vi "RecrystalliseSendAHKcmd.vi"(8 "error in (no error)":errorcluster, 11 "Enum":enum16{"low", "high"}(ring)) -> (0 "error out":errorcluster)   [LabVIEW 2017]
panel:
  out "timed out?":bool
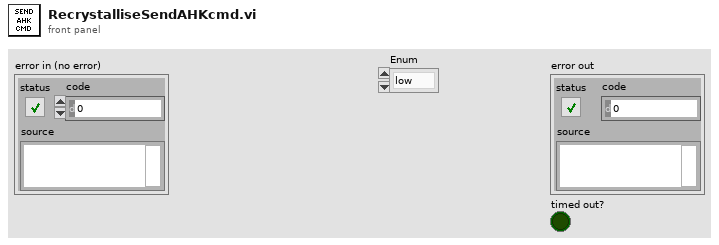
[diagram p1: front panel]
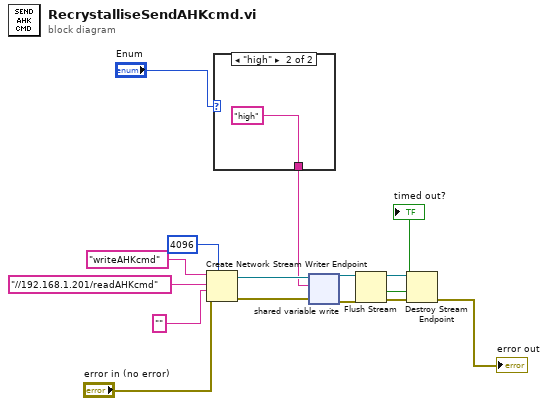
[diagram p0: block diagram]
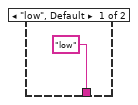
[diagram p2: hidden frame]
diagram:
  n1 = Create Network Stream Writer Endpoint(7:4096 ("writer buffer size"), 8:"error in (no error)", 9:"", 10:"//192.168.1.201/readAHKcmd" ("reader url"), 11:"writeAHKcmd" ("writer name")) -> (0:w10:errorcluster, 3:w11:refnum<k21>)  [unwired: 2 in]
  n2 = case shown="\"high\"" "Enum" {
    tunnel: ["low" ("data in") "high" ("data in")] -> w1
    frame "low", Default {
    }
    frame "high" {
    }
  }
  n3 = shared-variable-write(w11, w10, w1) -> (w5:refnum<k21>, w8:errorcluster)  [unwired: 1 in, 1 out]
  n4 = Flush Stream(8:w8, 11:w5) -> (0:w7:errorcluster, 1:→"timed out?":bool, 3:w6:refnum<k21>)  [unwired: 2 in]
  n5 = Destroy Stream Endpoint(8:w7, 11:w6) -> (0:→"error out":errorcluster)
